vi "GageSimpleConnexion.vi"() -> ()   [LabVIEW 2018]
panel:
  out "Handle Cluster":T1
  out "Number Of Systems":i32
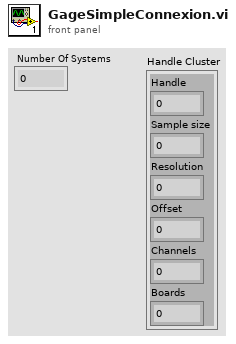
[diagram p1: front panel]
types:
  T1 = cluster{"Handle":u32, "Sample size":u32, "Resolution":i32, "Offset":i32, "Channels":u32, "Boards":u32}
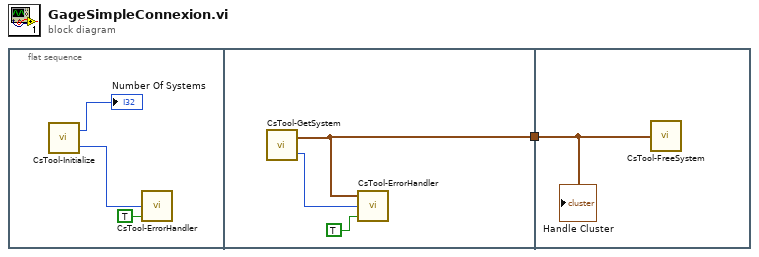
[diagram p0: block diagram]
diagram:
  n1 = flat-sequence {
    tunnel: [w5] -> w1
    tunnel: w1 -> [w8]
    frame #0 {
      n2 = call "CsTool-Initialize.vi"() -> ("Error Code"=w4:i32, "Number Of Systems"=→"Number Of Systems":i32)
      n3 = call "CsTool-ErrorHandler.vi"("StopOnError (true)"=TRUE, "Error Code"=w4) -> ()  [unwired: 1 in, 1 out]
    }
    frame #1 {
      n4 = call "CsTool-GetSystem.vi"() -> ("Error Code"=w6:i32, "Handle Cluster"=w5:T1)  [unwired: 4 in]
      n5 = call "CsTool-ErrorHandler.vi"("StopOnError (true)"=TRUE, "Error Code"=w6, "Handle Cluster"=w5) -> ()  [unwired: 1 out]
    }
    frame #2 {
      n6 = call "CsTool-FreeSystem.vi"("Handle Cluster"=w8) -> ()  [unwired: 1 out]
      "Handle Cluster" <- w8
    }
  }
